vi "Spin_Analysis.vi"(1 "路径 2":path, 2 "路径":path) -> (0 "ErrorInfo":string[](array[string]))   [LabVIEW 2011]
panel:
  out "TurnOFF":u32
  out "TurnON":u32
  out "FinalSpin_StepLoose":u32
  out "FinalStepSpinHoldingTime":u32
  out "FinalSpin_StepSpin":u32
  out "WaterLevel":i32
  out "FinalSpin_StepDrain":u32
  out "PROGRESS_FINALSPIN_Index":u32
  out "Initial_StepFirstDrain":u32
  out "Progress_INITIAL_Index":u32
  out "RUNMODE_RUNNING_Index":u32
  out "POWER_ON_Index":u32
  out "POWER_UPSTART_Index":u32
  out "EXCEL读取":string[][](array[string])
  out "FinalSpinEnd_Index":u32
  # "Spec比对文件路径"
  # "采集数据存储文件路径"
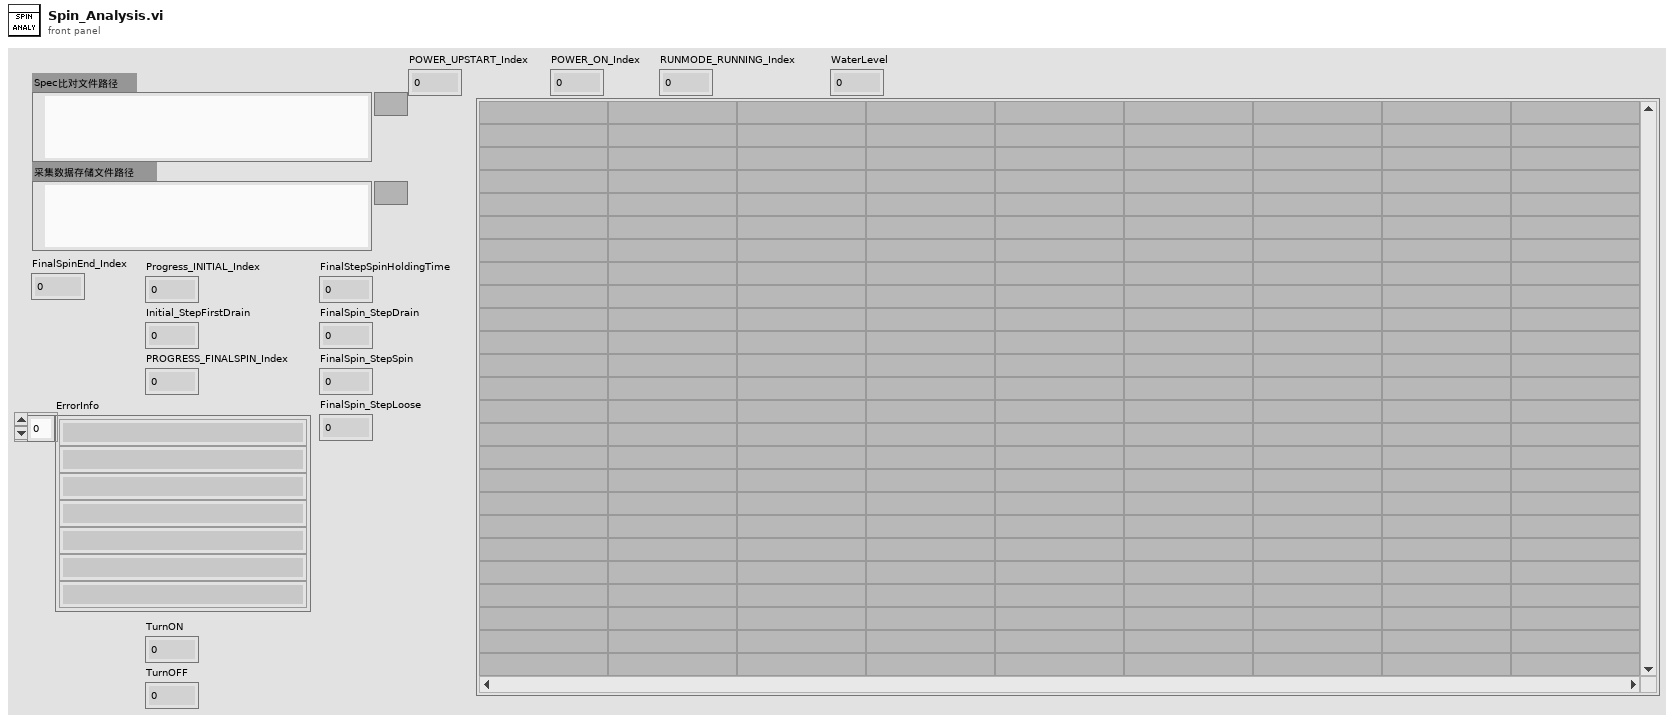
[diagram p1: front panel]
types:
  T1 = cluster{"FinalSpin_ArrayLength":u32, "FinalSpin_StepInit":u32, "FinalSpin_StepDrain":u32, "FinalSpin_StepSudsReduction":u32, "FinalSpin_StepSpin":u32, "FinalSpin_StepLoose":u32, "FinalSpin_StepEnd":u32, "PROGRESS_FINALSPIN_Index":u32}
  T2 = cluster{"RUNMODE_READY_Index":u32, "RUNMODE_RUNNING_Index":u32}
  T3 = cluster{"Initial_ArrayLength":u32, "Initial_StepInit":u32, "Initial_StepFirstDrainInitial":u32, "Initial_StepFirstDrain":u32, "Progress_INITIAL_Index":u32}
  T4 = cluster{"POWER_UPSTART_Index":u32, "POWER_ON_Index":u32}
  T5 = cluster{"Step1":cluster{"Speed":u32, "Time":u32}, "Step2":cluster{"Speed":u32, "Time":u32}, "Step3":cluster{"Speed":u32, "Time":u32}, "Untangle":cluster{"Speed":u32, "On":u32, "Off":u32}}
  T6 = cluster{"DrainTime":u32, "FinalSpinTime":u32, "LooseTime":u32, "SubTotalTime":u32}
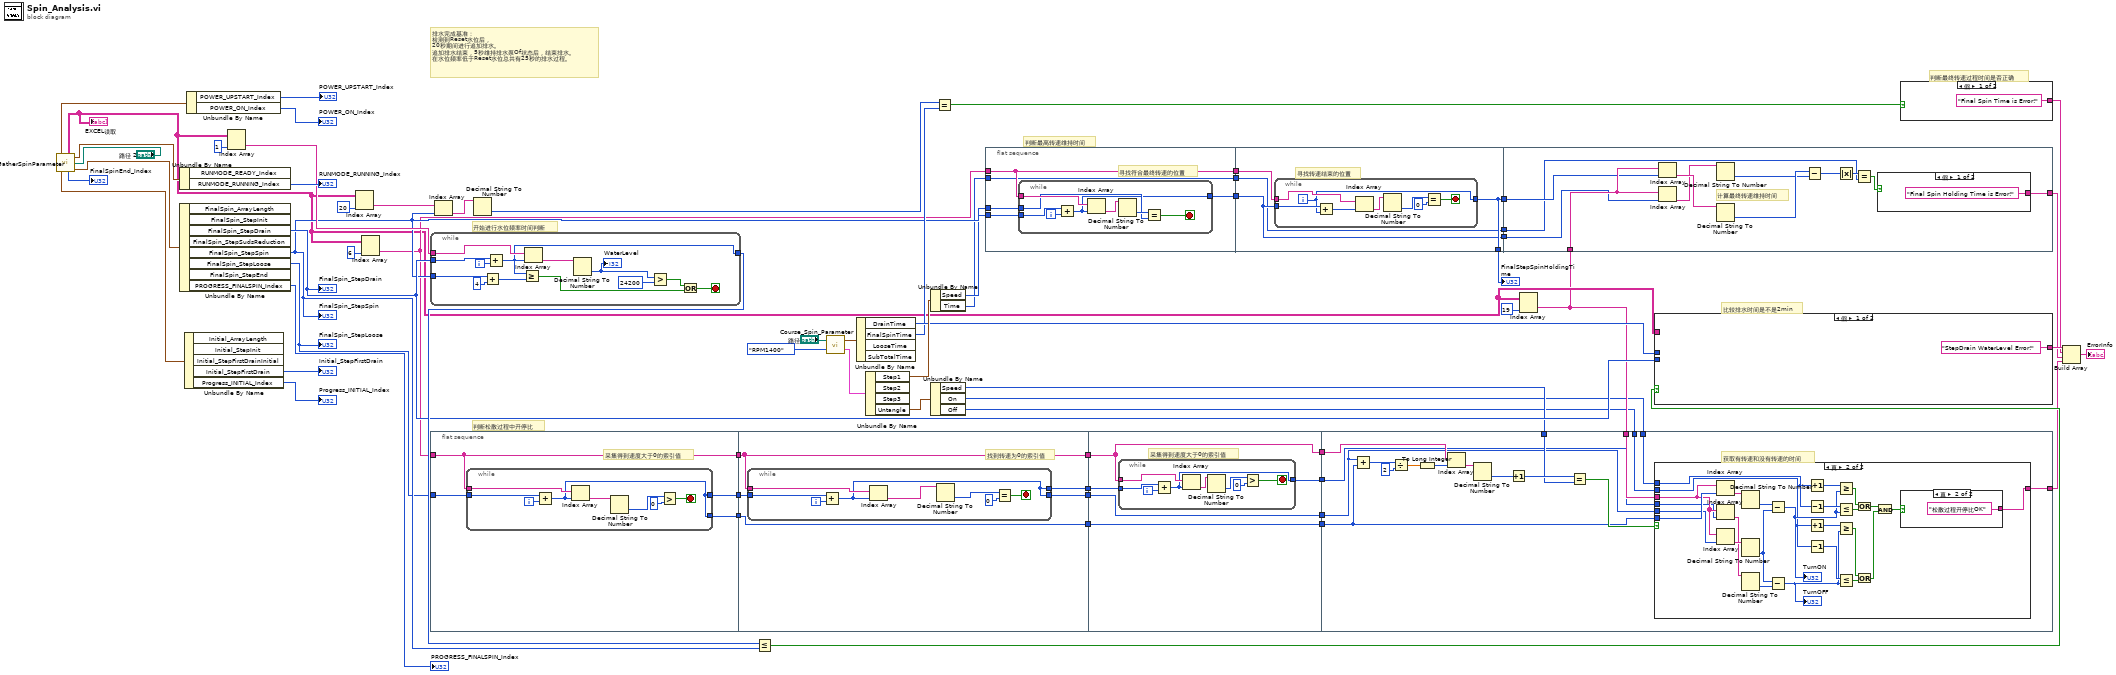
[diagram p0: block diagram]
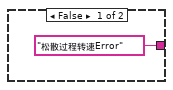
[diagram p2: hidden frame]
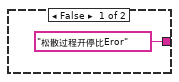
[diagram p3: hidden frame]
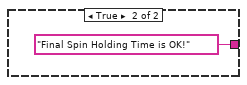
[diagram p4: hidden frame]
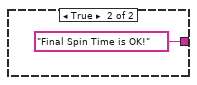
[diagram p5: hidden frame]
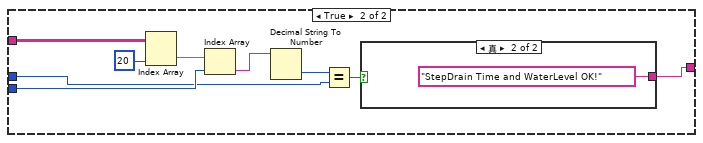
[diagram p6: hidden frame]
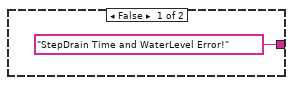
[diagram p7: hidden frame]
diagram:
  # "判断松散过程中开停比"
  # "判断最高转速维持时间"
  # "判断最终转速过程时间是否正确"
  # "比较排水时间是不是2min"
  # "开始进行水位频率时间判断"
  # "排水完成基准：\n检测到Reset水位后，\n20秒期间进行追加排水。\n追加排水结束，5秒维持排水泵Of状态后，结束排水。\n在水位频率低于Reset水位总共有25秒的排水过程。"
  n1 = call "GatherSpinParameter.vi"("路径"="路径 2") -> ("ProgressFinalSpin"=w58:T1, "FinalSpinEnd_Index"=→"FinalSpinEnd_Index":u32, "RUNStateID"=w57:T2, "EXCEL读取"=w6:string[][], "ProgressInitial"=w55:T3, "POWERStateID"=w56:T4)
  "EXCEL读取" <- w6
  n2 = Unbundle By Name(w57) -> ("RUNMODE_RUNNING_Index"=→"RUNMODE_RUNNING_Index":u32)  [unwired: 1 out]
  n3 = Unbundle By Name(w58) -> ("FinalSpin_StepDrain"=w43:u32, "FinalSpin_StepSpin"=w34:u32, "FinalSpin_StepLoose"=w18:u32, "PROGRESS_FINALSPIN_Index"=→"PROGRESS_FINALSPIN_Index":u32)  [unwired: 4 out]
  "FinalSpin_StepDrain" <- w43
  "FinalSpin_StepSpin" <- w34
  "FinalSpin_StepLoose" <- w18
  n4 = Unbundle By Name(w55) -> ("Initial_StepFirstDrain"=→"Initial_StepFirstDrain":u32, "Progress_INITIAL_Index"=→"Progress_INITIAL_Index":u32)  [unwired: 3 out]
  n5 = Unbundle By Name(w56) -> ("POWER_UPSTART_Index"=→"POWER_UPSTART_Index":u32, "POWER_ON_Index"=→"POWER_ON_Index":u32)
  n6 = Index Array(array=w6, index (col)=1 ("禁用的索引 (列)")) -> (element=w48:string[])  [unwired: 1 in]
  n7 = Index Array(array=w6, index (col)=20 ("禁用的索引 (列)")) -> (element=w40:string[])  [unwired: 1 in]
  n8 = Index Array(array=w6, index (col)=6 ("禁用的索引 (列)")) -> (element=w19:string[])  [unwired: 1 in]
  n9 = while {
    tunnel: w48 -> [w78]
    tunnel: w43 -> [w73]
    tunnel: [w70] -> w45
    tunnel: w34 -> [w68]
    i -> [w74]
    stop <- w71 stop-if-true
    n10 = Add(x=w68, y=u32 4) -> (x+y=w66:u32)
    n11 = Add(x=w73, y=w74) -> (x+y=w70:u32)
    n12 = Greater Or Equal?(x=w70, y=w66) -> (x >= y?=w69:bool)
    n13 = Index Array(array=w78, index=w70) -> (element=w77:string)
    n14 = Decimal String To Number(string=w77) -> (number=w75:i32)  [unwired: 2 in, 1 out]
    "WaterLevel" <- w75
    n15 = Greater?(x=w75, y=24200) -> (0:w72:bool)
    n16 = Or(x=w72, y=w69) -> (x .or. y?=w71:bool)
  }
  n17 = flat-sequence {
    tunnel: w19 -> [w81]
    tunnel: w18 -> [w82]
    tunnel: [w81] -> w17
    tunnel: [w80] -> w16
    tunnel: [w79] -> w10
    tunnel: w17 -> [w94]
    tunnel: w16 -> [w95]
    tunnel: [w94] -> w15
    tunnel: [w93] -> w14
    tunnel: [w92] -> w12
    tunnel: w10 -> [w91]
    tunnel: [w91] -> w9
    tunnel: w15 -> [w107]
    tunnel: w14 -> [w108]
    tunnel: [w107] -> w13
    tunnel: w12 -> [w106]
    tunnel: [w106] -> w11
    tunnel: w9 -> [w105]
    tunnel: [w105] -> w8
    tunnel: [w104] -> w4
    tunnel: w13 -> [w132]
    tunnel: w11 -> [w121]
    tunnel: w8 -> [w122]
    tunnel: w7 -> [w125]
    tunnel: w5 -> [w123]
    tunnel: w4 -> [w120]
    tunnel: w3 -> [w119]
    tunnel: w2 -> [w118]
    tunnel: [w117] -> w1
    frame #0 {
      # "采集得到速度大于0的索引值"
      n18 = while {
        tunnel: w81 -> [w90]
        tunnel: w82 -> [w89]
        tunnel: [w83] -> w80
        tunnel: [w83] -> w79
        i -> [w88]
        stop <- w84 stop-if-true
        n19 = Add(x=w89, y=w88) -> (x+y=w83:u32)
        n20 = Index Array(array=w90, index=w83) -> (element=w87:string)
        n21 = Decimal String To Number(string=w87) -> (number=w86:i32)  [unwired: 2 in, 1 out]
        n22 = Greater?(x=w86, y=0) -> (0:w84:bool)
      }
    }
    frame #1 {
      # "找到转速为0的索引值"
      n23 = while {
        tunnel: w94 -> [w103]
        tunnel: w95 -> [w101]
        tunnel: [w96] -> w92
        tunnel: [w96] -> w93
        i -> [w102]
        stop <- w97 stop-if-true
        n24 = Add(x=w101, y=w102) -> (x+y=w96:u32)
        n25 = Index Array(array=w103, index=w96) -> (element=w100:string)
        n26 = Decimal String To Number(string=w100) -> (number=w99:i32)  [unwired: 2 in, 1 out]
        n27 = Equal?(x=w99, y=0) -> (x = y?=w97:bool)
      }
    }
    frame #2 {
      # "采集得到速度大于0的索引值"
      n28 = while {
        tunnel: w107 -> [w116]
        tunnel: w108 -> [w115]
        tunnel: [w109] -> w104
        i -> [w114]
        stop <- w110 stop-if-true
        n29 = Add(x=w115, y=w114) -> (x+y=w109:u32)
        n30 = Index Array(array=w116, index=w109) -> (element=w113:string)
        n31 = Decimal String To Number(string=w113) -> (number=w112:i32)  [unwired: 2 in, 1 out]
        n32 = Greater?(x=w112, y=0) -> (0:w110:bool)
      }
    }
    frame #3 {
      # "获取有转速和没有转速的时间"
      n33 = Add(x=w121, y=w122) -> (x+y=w131:u32)
      n34 = Divide(x=w131, y=u32 2) -> (x/y=w129:dbl)
      n35 = To Long Integer(number=w129) -> (32bit integer=w128:i32)
      n36 = Index Array(array=w132, index=w128) -> (element=w133:string)
      n37 = Decimal String To Number(string=w133) -> (number=w127:i32)  [unwired: 2 in, 1 out]
      n38 = Increment(x=w127) -> (x+1=w126:i32)
      n39 = Equal?(x=w126, y=w125) -> (x = y?=w124:bool)
      n40 = case shown="真" w124 {
        tunnel: w123 -> [_ w156]
        tunnel: w122 -> [_ w160]
        tunnel: w121 -> [_ w159]
        tunnel: w120 -> [_ w155]
        tunnel: w119 -> [_ w148]
        tunnel: w118 -> [_ w139]
        tunnel: ["松散过程转速Error" w135] -> w117
        frame False {
        }
        frame True {
          n41 = Index Array(array=w156, index=w160) -> (element=w158:string)
          n42 = Index Array(array=w156, index=w155) -> (element=w154:string)
          n43 = Index Array(array=w156, index=w159) -> (element=w157:string)
          n44 = Decimal String To Number(string=w158) -> (number=w153:i32)  [unwired: 2 in, 1 out]
          n45 = Decimal String To Number(string=w157) -> (number=w152:i32)  [unwired: 2 in, 1 out]
          n46 = Decimal String To Number(string=w154) -> (number=w151:i32)  [unwired: 2 in, 1 out]
          n47 = Subtract(x=w153, y=w152) -> (x-y=w143:i32)
          "TurnON" <- w143
          n48 = Subtract(x=w152, y=w151) -> (x-y=w140:i32)
          "TurnOFF" <- w140
          n49 = Increment(x=w148) -> (x+1=w144:u32)
          n50 = Decrement(x=w148) -> (x-1=w145:u32)
          n51 = Increment(x=w139) -> (x+1=w142:u32)
          n52 = Decrement(x=w139) -> (x-1=w141:u32)
          n53 = Greater Or Equal?(x=w144, y=w143) -> (x >= y?=w150:bool)
          n54 = Less Or Equal?(x=w145, y=w143) -> (x <= y?=w149:bool)
          n55 = Greater Or Equal?(x=w142, y=w140) -> (x >= y?=w147:bool)
          n56 = Less Or Equal?(x=w141, y=w140) -> (x <= y?=w146:bool)
          n57 = Or(x=w150, y=w149) -> (x .or. y?=w138:bool)
          n58 = Or(x=w147, y=w146) -> (x .or. y?=w137:bool)
          n59 = And(x=w138, y=w137) -> (x .and. y?=w136:bool)
          n60 = case shown="真" w136 {
            tunnel: ["松散过程开停比Eror" "松散过程开停比OK"] -> w135
            frame False {
            }
            frame True {
            }
          }
        }
      }
    }
  }
  n61 = Index Array(array=w40, index=w34) -> (element=w39:string)
  n62 = Decimal String To Number(string=w39) -> (number=w38:i32)  [unwired: 2 in, 1 out]
  n63 = Less Or Equal?(x=w45, y=w34) -> (x <= y?=w44:bool)
  n64 = call "Course_Spin_Parameter.vi"("RpmOptionChoose"=enum16{"RPM1400", "RPM1600"}."RPM1400", "路径"="路径") -> ("SpeedTime"=w62:T5, "PrjFinalSpinTime"=w63:T6)
  n65 = Unbundle By Name(w63) -> ("DrainTime"=w42:u32, "FinalSpinTime"=w37:u32)  [unwired: 2 out]
  n66 = Unbundle By Name(w62) -> ("Step1"=w61:cluster{"Speed":u32, "Time":u32}, "Untangle"=w60:cluster{"Speed":u32, "On":u32, "Off":u32})  [unwired: 2 out]
  n67 = Unbundle By Name(w61) -> ("Speed"=w33:u32, "Time"=w26:u32)
  n68 = Unbundle By Name(w60) -> ("Speed"=w7:u32, "On"=w3:u32, "Off"=w2:u32)
  n69 = Equal?(x=w38, y=w37) -> (x = y?=w36:bool)
  n70 = flat-sequence {
    tunnel: w19 -> [w165]
    tunnel: w34 -> [w167]
    tunnel: w33 -> [w166]
    tunnel: [w165] -> w32
    tunnel: [w164] -> w31
    tunnel: w26 -> [w163]
    tunnel: [w163] -> w25
    tunnel: w32 -> [w179]
    tunnel: w31 -> [w177]
    tunnel: [w178] -> w30
    tunnel: [w178] -> w28
    tunnel: [w177] -> w27
    tunnel: w25 -> [w176]
    tunnel: [w176] -> w24
    tunnel: w5 -> [w199]
    tunnel: w28 -> [w198]
    tunnel: w27 -> [w197]
    tunnel: w24 -> [w190]
    tunnel: [w188] -> w21
    frame #0 {
      # "寻找符合最终转速的位置"
      n71 = while {
        tunnel: w165 -> [w175]
        tunnel: w167 -> [w173]
        tunnel: w166 -> [w170]
        tunnel: [w168] -> w164
        i -> [w174]
        stop <- w169 stop-if-true
        n72 = Add(x=w173, y=w174) -> (x+y=w168:u32)
        n73 = Index Array(array=w175, index=w168) -> (element=w172:string)
        n74 = Decimal String To Number(string=w172) -> (number=w171:i32)  [unwired: 2 in, 1 out]
        n75 = Equal?(x=w171, y=w170) -> (x = y?=w169:bool)
      }
    }
    frame #1 {
      # "寻找转速结束的位置"
      n76 = while {
        tunnel: w179 -> [w187]
        tunnel: w177 -> [w186]
        tunnel: [w181] -> w178
        i -> [w181]
        stop <- w182 stop-if-true
        n77 = Add(x=w186, y=w181) -> (x+y=w180:u32)
        n78 = Index Array(array=w187, index=w180) -> (element=w185:string)
        n79 = Decimal String To Number(string=w185) -> (number=w184:i32)  [unwired: 2 in, 1 out]
        n80 = Equal?(x=w184, y=0) -> (x = y?=w182:bool)
      }
    }
    frame #2 {
      # "计算最终转速维持时间"
      n81 = Index Array(array=w199, index=w198) -> (element=w196:string)
      n82 = Index Array(array=w199, index=w197) -> (element=w195:string)
      n83 = Decimal String To Number(string=w195) -> (number=w193:i32)  [unwired: 2 in, 1 out]
      n84 = Decimal String To Number(string=w196) -> (number=w194:i32)  [unwired: 2 in, 1 out]
      n85 = Subtract(x=w194, y=w193) -> (x-y=w192:i32)
      n86 = Absolute Value(x=w192) -> (abs(x)=w191:i32)
      n87 = Equal?(x=w191, y=w190) -> (x = y?=w189:bool)
      n88 = case shown="假" w189 {
        tunnel: ["Final Spin Holding Time is Error!" ("消息") "Final Spin Holding Time is OK!" ("消息")] -> w188
        frame False {
        }
        frame True {
        }
      }
    }
  }
  n89 = Index Array(array=w6, index (col)=19 ("禁用的索引 (列)")) -> (element=w5:string[])  [unwired: 1 in]
  n90 = case shown="假" w44 {
    tunnel: w6 -> [_ w211]
    tunnel: w43 -> [_ w208]
    tunnel: w42 -> [_ w204]
    tunnel: ["StepDrain WaterLevel Error!" ("消息") w203] -> w23
    frame False {
    }
    frame True {
      n91 = Index Array(array=w211, index (col)=20 ("禁用的索引 (列)")) -> (element=w209:string[])  [unwired: 1 in]
      n92 = Index Array(array=w209, index=w208) -> (element=w207:string)
      n93 = Decimal String To Number(string=w207) -> (number=w206:i32)  [unwired: 2 in, 1 out]
      n94 = Equal?(x=w206, y=w204) -> (x = y?=w205:bool)
      n95 = case shown="真" w205 {
        tunnel: ["StepDrain Time and WaterLevel Error!" ("消息") "StepDrain Time and WaterLevel OK!" ("消息")] -> w203
        frame False {
        }
        frame True {
        }
      }
    }
  }
  n96 = case shown="假" w36 {
    tunnel: ["Final Spin Time is Error!" ("消息") "Final Spin Time is OK!" ("消息")] -> w22
    frame False {
    }
    frame True {
    }
  }
  n97 = Build Array(w23, w22, w21, w1) -> (→"ErrorInfo":string[])
  "FinalStepSpinHoldingTime" <- w30
